vi "Start.vi"(7 "ConcreteActor":refnum<class "ConcreteActor.lvclass">) -> (5 "ConcreteActor":refnum<class "ConcreteActor.lvclass">)   [LabVIEW 2020, in "_Template.lvlib" / "ActorTemplate.lvlib" / "{{Name}}.lvlib" / "ConcreteActor.lvclass"]
uses:
  ConcreteActor.lvclass
  ConcreteActor.lvclass/ConcreteActor.ctl
  jettl/jettl/Actor/Actor.lvclass
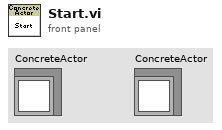
[diagram p1: front panel]
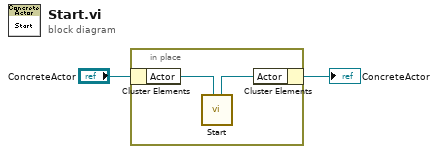
[diagram p0: block diagram]
diagram:
  n1 = in-place {
    n2 = in-place-cluster #1("ConcreteActor") -> ("Actor"=w3:refnum<class "Actor.lvclass">)
    n3 = call-dynamic "Start.vi"("Actor"=w3) -> ("Actor"=w4:refnum<class "Actor.lvclass">)  [unwired: 10 in]
    n4 = in-place-cluster #1("Actor"=w4) -> (→"ConcreteActor":refnum<class "ConcreteActor.lvclass">)
  }
